vi "Write Default Path Cluster.vi"(8 "error in (no error)":errorcluster, 10 "Default Path":T1, 11 "Path Settings in":refnum<class "Path Settings.lvclass">) -> (0 "error out":errorcluster, 3 "Path Settings out":refnum<class "Path Settings.lvclass">)   [LabVIEW 2019, in "Path Settings.lvclass"]
uses:
  Path Settings.lvclass
  Default Path Cluster.ctl
  Path Settings.lvclass/Path Settings.ctl
  <vilib>/JDP Science/JSONtext/JSONtext.lvlib
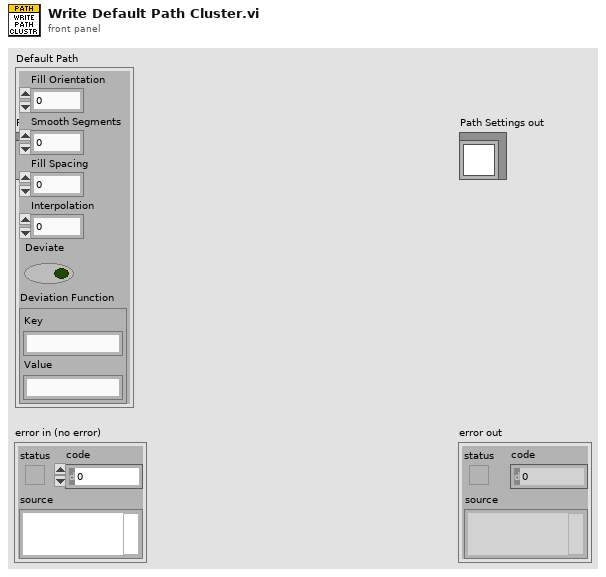
[diagram p1: front panel]
types:
  T1 = typedef "Path Settings.lvclass/Default Path Cluster.ctl" = cluster{"Fill Orientation":u16, "Smooth Segments":dbl, "Fill Spacing":dbl, "Interpolation":dbl, "Deviate":bool, "Deviation Function":cluster{"Key":string, "Value":string}}
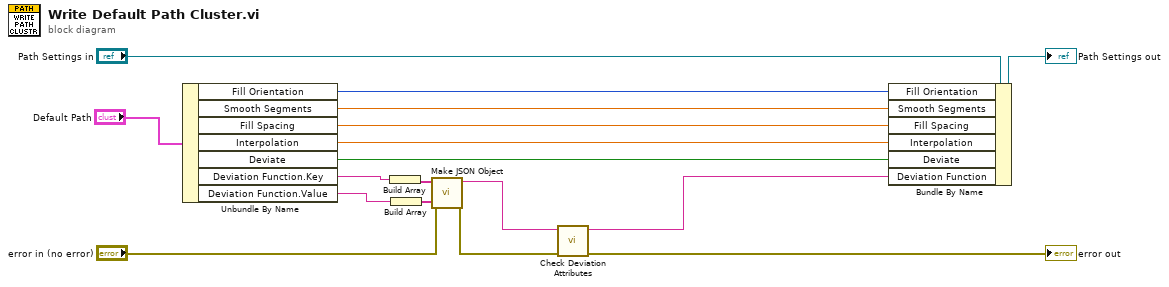
[diagram p0: block diagram]
diagram:
  n1 = Unbundle By Name("Default Path") -> ("Fill Orientation"=w14:u16, "Smooth Segments"=w13:dbl, "Fill Spacing"=w12:dbl, "Interpolation"=w11:dbl, "Deviate"=w10:bool, "Deviation Function.Key"=w7:string, "Deviation Function.Value"=w6:string)
  n2 = Build Array(w7) -> (w5:string[])
  n3 = Build Array(w6) -> (w4:string[])
  n4 = call <vilib>:"Make JSON Object.vi"("error in (no error)"="error in (no error)", "JSON Items"=w4, "Item Names"=w5) -> ("error out"=w1:errorcluster, "<JSON>"=w3:string)  [unwired: 7 in]
  n5 = call "Check Deviation Attributes.vi"("error in (no error)"=w1, "Deviation In"=w3) -> ("error out"=→"error out":errorcluster, "Deviation Out"=w9:string)  [unwired: 8 in]
  n6 = Bundle By Name(cluster="Path Settings in", "Fill Orientation"=w14, "Smooth Segments"=w13, "Fill Spacing"=w12, "Interpolation"=w11, "Deviate"=w10, "Deviation Function"=w9) -> (→"Path Settings out":refnum<class "Path Settings.lvclass">)
